vi "NOx MFR age.vi"(9 "NOx conc":dbl=0.1, 10 "NOx PV":dbl, 11 "Flow rate l/min":dbl) -> (3 "NOx MFR":dbl)   [LabVIEW 2011]
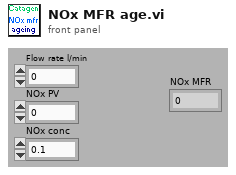
[diagram p1: front panel]
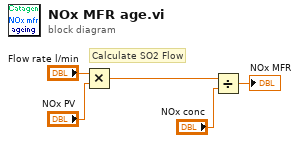
[diagram p0: block diagram]
diagram:
  # "Calculate SO2 Flow"
  n1 = Multiply(x="Flow rate l/min", y="NOx PV") -> (x*y=w1:dbl)
  n2 = Divide(x=w1, y="NOx conc") -> (x/y=→"NOx MFR":dbl)
